vi "CheckVoltageMagnitude.vi"(9 "nominal line voltage":dbl, 10 "Wiring Configuration":string, 11 "voltage phasors":cdb[](array[numeric])) -> (2 "wiring info":string, 3 "valid?":bool)   [LabVIEW 2017, in "McsaAnalysisLowRate.lvlib"]
uses:
  <vilib>/addons/InsightCM/Devices/Shared/Mcsa/McsaAnalysisLowRate/McsaAnalysisLowRate.lvlib
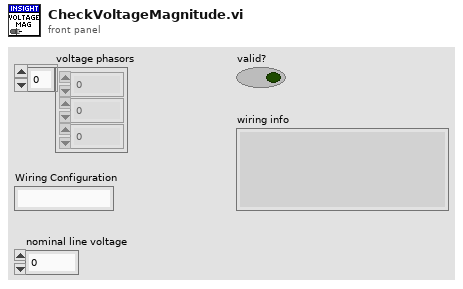
[diagram p1: front panel]
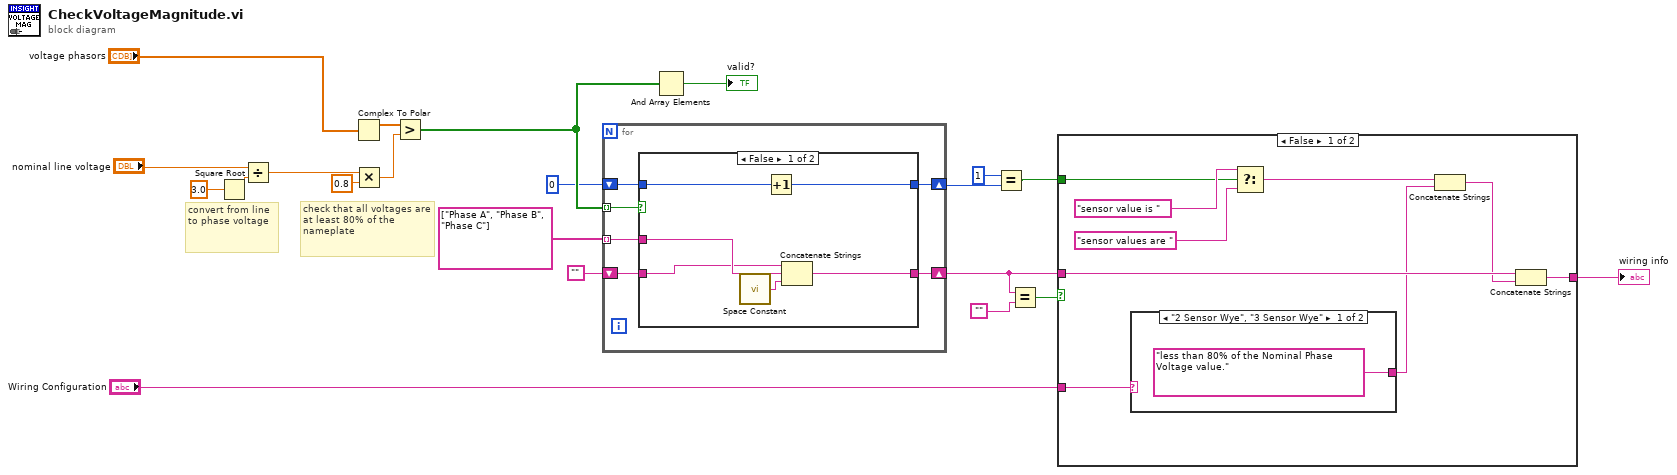
[diagram p0: block diagram]
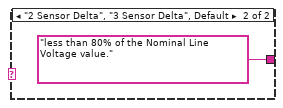
[diagram p2: hidden frame]
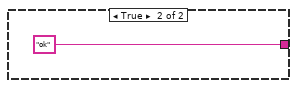
[diagram p3: hidden frame]
diagram:
  # "convert from line to phase voltage"
  # "check that all voltages are at least 80% of the nameplate"
  n1 = Square Root(x=3.0) -> (sqrt(x)=w2:dbl)
  n2 = Divide(x="nominal line voltage", y=w2) -> (x/y=w19:dbl)
  n3 = Complex To Polar(r * e^(i*theta)="voltage phasors") -> (r=w15:dbl[])  [unwired: 1 out]
  n4 = Multiply(x=w19, y=0.8) -> (x*y=w16:dbl)
  n5 = Greater?(x=w15, y=w16) -> (0:w13:bool[])
  n6 = for {
    tunnel: string[] ["Phase A", "Phase B", "Phase C"] -> [w25] mode=indexing
    shift-right: [w26] -> w10
    shift-left: "" -> [w27]
    tunnel: w13 -> [w24] mode=indexing
    shift-right: [w23] -> w7
    shift-left: 0 -> [w22]
    n7 = case shown="False" w24 {
      tunnel: w27 -> [w31 w35]
      tunnel: [w33 w35] -> w26
      tunnel: w25 -> [w32 _]
      tunnel: [w29 w34] -> w23
      tunnel: w22 -> [w30 w34]
      frame False {
        n8 = call <vilib>:"Space Constant.vi"() -> ("String"=w28:string)
        n9 = Increment(x=w30) -> (x+1=w29:i32)
        n10 = Concatenate Strings(w31, w32, w28) -> (w33:string)
      }
      frame True {
      }
    }
  }
  n11 = And Array Elements(Boolean array=w13) -> (logical AND=→"valid?":bool)
  n12 = Equal?(x=1, y=w7) -> (x = y?=w5:bool)
  n13 = Equal?(x=w10, y="") -> (x = y?=w11:bool)
  n14 = case shown="False" w11 {
    tunnel: w10 -> [w43 _]
    tunnel: [w42 "ok"] -> w12
    tunnel: w5 -> [w40 _]
    tunnel: "Wiring Configuration" -> [w36 _]
    frame False {
      n15 = case shown="\"2 Sensor Wye\", \"3 Sensor Wye\"" w36 {
        tunnel: ["less than 80% of the Nominal Phase Voltage value." "less than 80% of the Nominal Line Voltage value."] -> w37
        frame "2 Sensor Wye", "3 Sensor Wye" {
        }
        frame "2 Sensor Delta", "3 Sensor Delta", Default {
        }
      }
      n16 = Select(t="sensor value is ", s=w40, f="sensor values are ") -> (s? t:f=w39:string)
      n17 = Concatenate Strings(w39, w37) -> (w38:string)
      n18 = Concatenate Strings(w43, w38) -> (w42:string)
    }
    frame True {
    }
  }
  "wiring info" <- w12
